vi "getPosition-Old-Controllers.vi"(2 "Motor (XYZ)":string(combo)="X", 3 "Device":refnum<k24>) -> (1 "GetPOS":dbl)   [LabVIEW 2014]
doc: "André Romero - 2017\nandretec@ifsc.usp.br"
uses:
  C:/UserLabs/Andre/LabView2014-32bits/kinesisTec/Kinesis/Thorlabs.MotionControl.TCube.DCServoCLI.dll
  Kinesis/Thorlabs.MotionControl.TCube.DCServoCLI.dll
  motor-XYZ-GlobalVar.vi
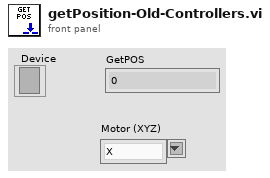
[diagram p1: front panel]
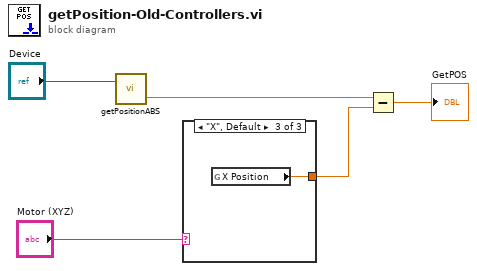
[diagram p0: block diagram]
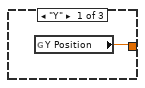
[diagram p2: hidden frame]
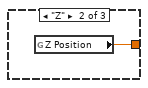
[diagram p3: hidden frame]
diagram:
  n1 = call "getPositionABS.vi"("Device"="Device") -> ("GetPOS"=w3:dbl)  [unwired: 1 in, 1 out]
  n2 = case shown="\"X\", Default" "Motor (XYZ)" {
    tunnel: [w6 w7 w8] -> w2
    frame "Y" {
      n3 = global read "motor-XYZ-GlobalVar.vi" "Y Position"() -> (w6:dbl)
    }
    frame "Z" {
      n4 = global read "motor-XYZ-GlobalVar.vi" "Z Position"() -> (w7:dbl)
    }
    frame "X", Default {
      n5 = global read "motor-XYZ-GlobalVar.vi" "X Position"() -> (w8:dbl)
    }
  }
  n6 = Subtract(x=w3, y=w2) -> (x-y=→"GetPOS":dbl)
